vi "MotionProfileGeneratorFilter1Sum.vi"(1 "fl1":dbl, 2 "Input":bool, 3 "Previous Filter1Sum":dbl) -> (0 "Filter1Sum":dbl)   [LabVIEW 2017]
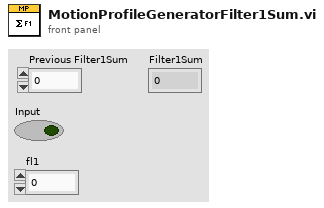
[diagram p1: front panel]
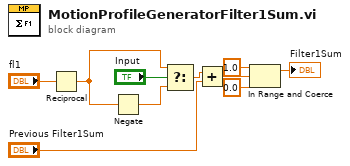
[diagram p0: block diagram]
diagram:
  n1 = Reciprocal(x="fl1") -> (1/x=w4:dbl)
  n2 = Negate(x=w4) -> (-x=w5:dbl)
  n3 = Select(t=w4, s="Input", f=w5) -> (s? t:f=w8:dbl)
  n4 = Add(x=w8, y="Previous Filter1Sum") -> (x+y=w7:dbl)
  n5 = In Range and Coerce(upper limit=1.0, x=w7, lower limit=0.0) -> (coerced(x)=→"Filter1Sum":dbl)  [unwired: 1 out]
